vi "Calculate Compas.vi"(11 "Gyro Angle":dbl) -> (3 "Compase reading":dbl)   [LabVIEW 2017]
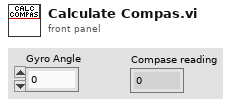
[diagram p1: front panel]
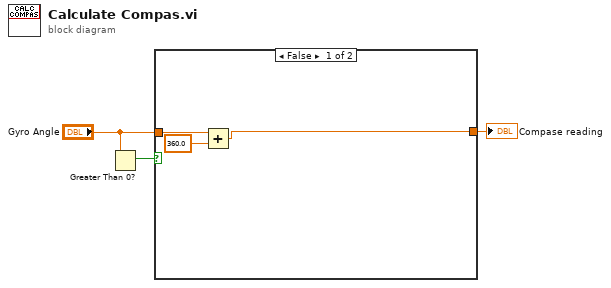
[diagram p0: block diagram]
diagram:
  n1 = Greater Than 0?(x="Gyro Angle") -> (x > 0?=w3:bool)
  n2 = case shown="False" w3 {
    tunnel: "Gyro Angle" -> [w6 w7]
    tunnel: [w4 w7] -> w1
    frame False {
      n3 = Add(x=w6, y=360.0) -> (x+y=w4:dbl)
    }
    frame True {
    }
  }
  "Compase reading" <- w1
